vi "ConvertData2.vi"(8 "error in (no error)":errorcluster, 11 "recordset data":variant[][](array[variant])) -> (0 "error out":errorcluster, 3 "Array":T1[](array[typedef]) {"SR#" format="%#_10g"})   [LabVIEW 2017, in "Server.lvlib" / "Oracle.lvlib"]
uses:
  Oracle.lvlib
  TypeDefs/SR Data.ctl
  <vilib>/addons/database/_DB Variant To Data/Database Variant To Data.xnode
  Server.lvlib
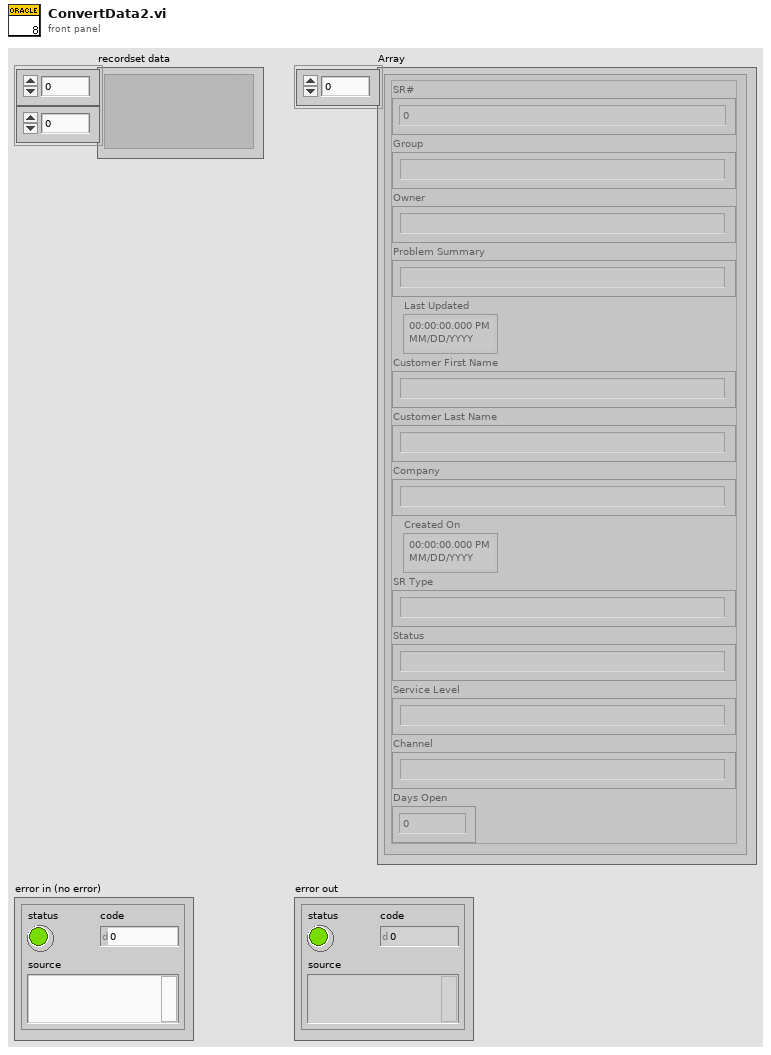
[diagram p1: front panel]
types:
  T1 = typedef "Server.lvlib/SR Data.ctl" = cluster{"SR#":dbl, "Group":string, "Owner":string, "Problem Summary":string, "Last Updated":timestamp, "Customer First Name":string, "Customer Last Name":string, "Company":string, "Created On":timestamp, "SR Type":string, "Status":string, "Service Level":string, "Channel":string, "Days Open":dbl}
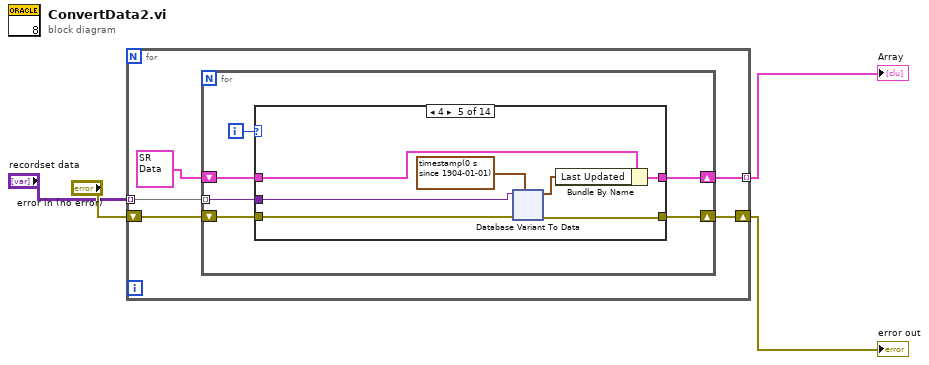
[diagram p0: block diagram]
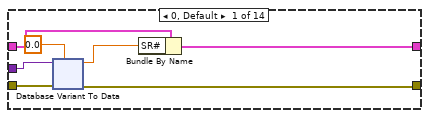
[diagram p2: hidden frame]
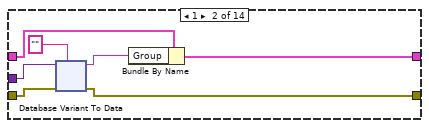
[diagram p3: hidden frame]
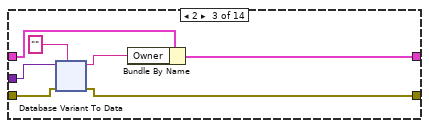
[diagram p4: hidden frame]
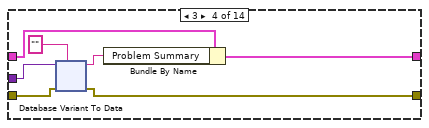
[diagram p5: hidden frame]
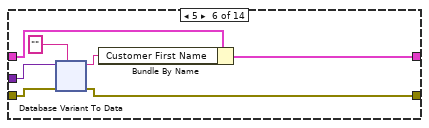
[diagram p6: hidden frame]
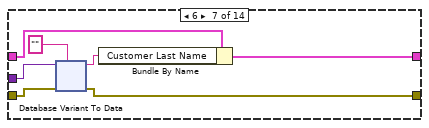
[diagram p7: hidden frame]
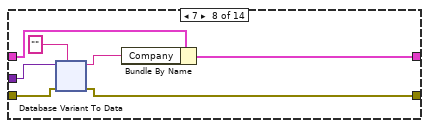
[diagram p8: hidden frame]
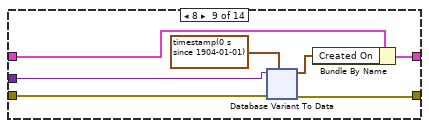
[diagram p9: hidden frame]
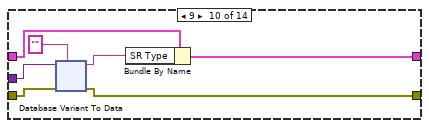
[diagram p10: hidden frame]
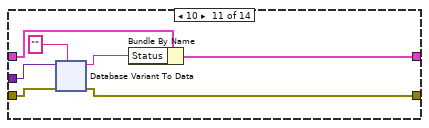
[diagram p11: hidden frame]
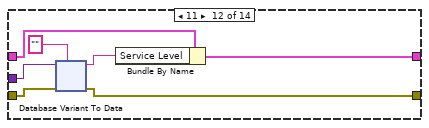
[diagram p12: hidden frame]
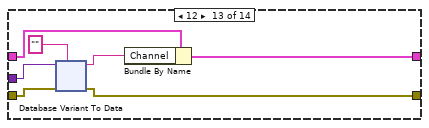
[diagram p13: hidden frame]
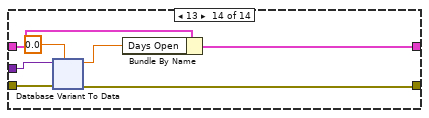
[diagram p14: hidden frame]
diagram:
  n1 = for {
    tunnel: "recordset data" -> [w9] mode=indexing
    tunnel: [w8] -> w1 mode=indexing
    shift-right: [w5] -> w4
    shift-left: "error in (no error)" -> [w6]
    n2 = for {
      tunnel: w9 -> [w14] mode=indexing
      shift-right: [w12] -> w8
      shift-left: T1 {"SR#"=0.0, "Group"="", "Owner"="", "Problem Summary"="", "Last Updated"=timestamp(0 s since 1904-01-01), "Customer First Name"="", "Customer Last Name"="", "Company"="", "Created On"=timestamp(0 s since 1904-01-01), "SR Type"="", "Status"="", "Service Level"="", "Channel"="", "Days Open"=0.0} ("SR Data") -> [w13]
      shift-right: [w10] -> w5
      shift-left: w6 -> [w11]
      i -> [w15]
      n3 = case shown="4" w15 {
        tunnel: w14 -> [w20 w60 w99 w138 w178 w229 w268 w307 w347 w398 w437 w476 w515 w553]
        tunnel: w13 -> [w22 w59 w98 w137 w176 w228 w267 w306 w345 w397 w436 w475 w514 w555]
        tunnel: [w18 w57 w96 w135 w175 w226 w265 w304 w344 w395 w434 w473 w512 w551] -> w12
        tunnel: w11 -> [w17 w56 w95 w134 w173 w225 w264 w303 w342 w394 w433 w472 w511 w550]
        tunnel: [w16 w55 w94 w133 w172 w224 w263 w302 w341 w393 w432 w471 w510 w549] -> w10
        frame 0, Default {
          n4 = xnode "Database Variant To Data"("database variant"=w20, "error in (no error)"=w17, "type"=0.0) -> ("data"=w19:dbl, "error out"=w16:errorcluster)
          n5 = Bundle By Name(cluster=w22, "SR#"=w19) -> (w18:T1)
        }
        frame 1 {
          n6 = xnode "Database Variant To Data"("database variant"=w60, "error in (no error)"=w56, "type"="" ("String")) -> ("data"=w58:string, "error out"=w55:errorcluster)
          n7 = Bundle By Name(cluster=w59, "Group"=w58) -> (w57:T1)
        }
        frame 2 {
          n8 = xnode "Database Variant To Data"("database variant"=w99, "error in (no error)"=w95, "type"="" ("String")) -> ("data"=w97:string, "error out"=w94:errorcluster)
          n9 = Bundle By Name(cluster=w98, "Owner"=w97) -> (w96:T1)
        }
        frame 3 {
          n10 = xnode "Database Variant To Data"("database variant"=w138, "error in (no error)"=w134, "type"="" ("String")) -> ("data"=w136:string, "error out"=w133:errorcluster)
          n11 = Bundle By Name(cluster=w137, "Problem Summary"=w136) -> (w135:T1)
        }
        frame 4 {
          n12 = xnode "Database Variant To Data"("database variant"=w178, "error in (no error)"=w173, "type"=timestamp(0 s since 1904-01-01)) -> ("data"=w174:timestamp, "error out"=w172:errorcluster)
          n13 = Bundle By Name(cluster=w176, "Last Updated"=w174) -> (w175:T1)
        }
        frame 5 {
          n14 = xnode "Database Variant To Data"("database variant"=w229, "error in (no error)"=w225, "type"="" ("String")) -> ("data"=w227:string, "error out"=w224:errorcluster)
          n15 = Bundle By Name(cluster=w228, "Customer First Name"=w227) -> (w226:T1)
        }
        frame 6 {
          n16 = xnode "Database Variant To Data"("database variant"=w268, "error in (no error)"=w264, "type"="" ("String")) -> ("data"=w266:string, "error out"=w263:errorcluster)
          n17 = Bundle By Name(cluster=w267, "Customer Last Name"=w266) -> (w265:T1)
        }
        frame 7 {
          n18 = xnode "Database Variant To Data"("database variant"=w307, "error in (no error)"=w303, "type"="" ("String")) -> ("data"=w305:string, "error out"=w302:errorcluster)
          n19 = Bundle By Name(cluster=w306, "Company"=w305) -> (w304:T1)
        }
        frame 8 {
          n20 = xnode "Database Variant To Data"("database variant"=w347, "error in (no error)"=w342, "type"=timestamp(0 s since 1904-01-01)) -> ("data"=w343:timestamp, "error out"=w341:errorcluster)
          n21 = Bundle By Name(cluster=w345, "Created On"=w343) -> (w344:T1)
        }
        frame 9 {
          n22 = xnode "Database Variant To Data"("database variant"=w398, "error in (no error)"=w394, "type"="" ("String")) -> ("data"=w396:string, "error out"=w393:errorcluster)
          n23 = Bundle By Name(cluster=w397, "SR Type"=w396) -> (w395:T1)
        }
        frame 10 {
          n24 = xnode "Database Variant To Data"("database variant"=w437, "error in (no error)"=w433, "type"="" ("String")) -> ("data"=w435:string, "error out"=w432:errorcluster)
          n25 = Bundle By Name(cluster=w436, "Status"=w435) -> (w434:T1)
        }
        frame 11 {
          n26 = xnode "Database Variant To Data"("database variant"=w476, "error in (no error)"=w472, "type"="" ("String")) -> ("data"=w474:string, "error out"=w471:errorcluster)
          n27 = Bundle By Name(cluster=w475, "Service Level"=w474) -> (w473:T1)
        }
        frame 12 {
          n28 = xnode "Database Variant To Data"("database variant"=w515, "error in (no error)"=w511, "type"="" ("String")) -> ("data"=w513:string, "error out"=w510:errorcluster)
          n29 = Bundle By Name(cluster=w514, "Channel"=w513) -> (w512:T1)
        }
        frame 13 {
          n30 = xnode "Database Variant To Data"("database variant"=w553, "error in (no error)"=w550, "type"=0.0) -> ("data"=w552:dbl, "error out"=w549:errorcluster)
          n31 = Bundle By Name(cluster=w555, "Days Open"=w552) -> (w551:T1)
        }
      }
    }
  }
  "error out" <- w4
  "Array" <- w1
